vi "AlliGator Harmonic Decomposition_Reorder Lifetimes & Fractions.vi"(0 "Reduced Lifetime 1":dbl, 5 "Fraction 1":dbl, 7 "Reduced Lifetime 2":dbl, 9 "Fraction 2":dbl, 11 "Error In":errorcluster) -> (4 "Smallest Reduced Lifetime (1)":dbl, 6 "Fraction 1":dbl, 8 "Largest Reduced Lifetime (2)":dbl, 10 "Fraction 2":dbl, 15 "Error Out":errorcluster)   [LabVIEW 2021, in "AlliGator Phasor Harmonics.lvlib"]
uses:
  AlliGator Phasor Harmonics.lvlib
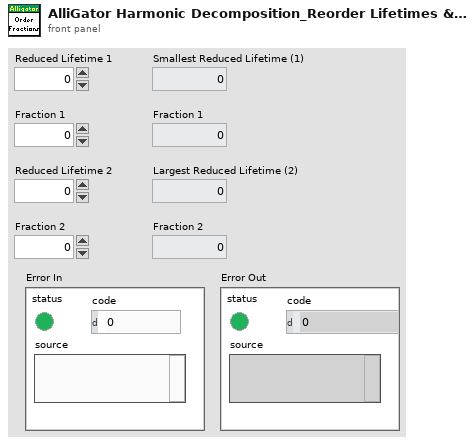
[diagram p1: front panel]
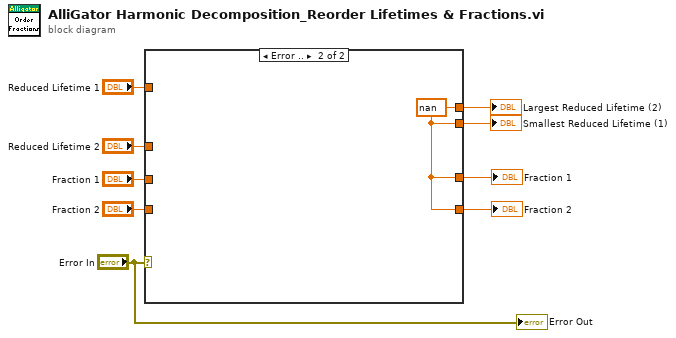
[diagram p0: block diagram]
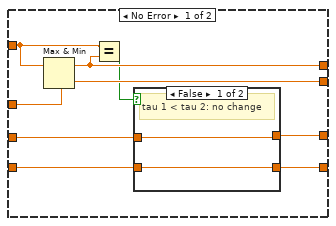
[diagram p2: hidden frame]
diagram:
  n1 = case shown="Error .." "Error In" {
    tunnel: "Reduced Lifetime 2" -> [w18 _]
    tunnel: [w17 w23] -> w8
    tunnel: "Reduced Lifetime 1" -> [w16 _]
    tunnel: [w15 w23] -> w6
    tunnel: "Fraction 1" -> [w13 _]
    tunnel: [w12 w23] -> w4
    tunnel: [w11 w23] -> w3
    tunnel: "Fraction 2" -> [w10 _]
    frame No Error {
      n2 = Max & Min(x=w16, y=w18) -> (max(x,y)=w15:dbl, min(x,y)=w17:dbl)
      n3 = Equal?(x=w16, y=w15) -> (x = y?=w14:bool)
      n4 = case shown="False" w14 {
        tunnel: w13 -> [w20 w22]
        tunnel: [w19 w22] -> w12
        tunnel: [w20 w21] -> w11
        tunnel: w10 -> [w19 w21]
        frame False {
          # "tau 1 < tau 2: no change"
        }
        frame True {
          # "tau 1 > tau 2: swap"
        }
      }
    }
    frame Error {
      w23 = nan
    }
  }
  "Fraction 1" <- w3
  "Fraction 2" <- w4
  "Largest Reduced Lifetime (2)" <- w6
  "Smallest Reduced Lifetime (1)" <- w8
  "Error Out" <- "Error In"
